vi "Expressions Example.vi"() -> ()   [LabVIEW 2022 SP3]
uses:
  Expressions/Expressions.lvlib
panel:
  out "error out":errorcluster
  in  "Expression":string(combo)="(a + b) * a - (c / b)"
  in  "f":bool=TRUE
  in  "e":bool
  in  "d":bool=TRUE
  in  "c":i32=-123
  in  "b":dbl=4.34
  in  "a":dbl=1.23
  out "Evaluated":dbl
  # "Instructions:\nEdit the Expression and run this VI to see the Evaluated result."
  # "The Expression statements are evaluated at run time.\nExpressions are first tokenized, parsed to postfix operations, then evaluated.\nAn expression can be nested in parentheses and consist of one or more operations,\nliterals, and/or variables. Supports either numerical expressions: (a + b * c) or \nboolean/conditional expressions: (a >= b or not c)."
  # "E.g. Numerical expression:    (a + b) * c"
  # "E.g. Boolean expression:    (d or e) and f"
  # "Variables"
  # "Supports:\nAND:          and | && | &\nOR:           or | '||' | '|'\nNOT:          not | !\nEQUAL:        ==\nNOT EQUAL:    !=\nLESS THAN:    <\nGREATER THAN: >\nLTE:          <=\nGTE:          >=\nPLUS:         +\nMINUS:        -\nMULTIPLY:     *\nDIVIDE:       /\nMODULUS:      %\nPARENTHESES:  (..)\nLITERAL:      Boolean | DBL | I32 | U32\nVARIABLE:    [A-Za-z_][A-Za-z0-9_]*\n  Note: Variables are referenced by name index."
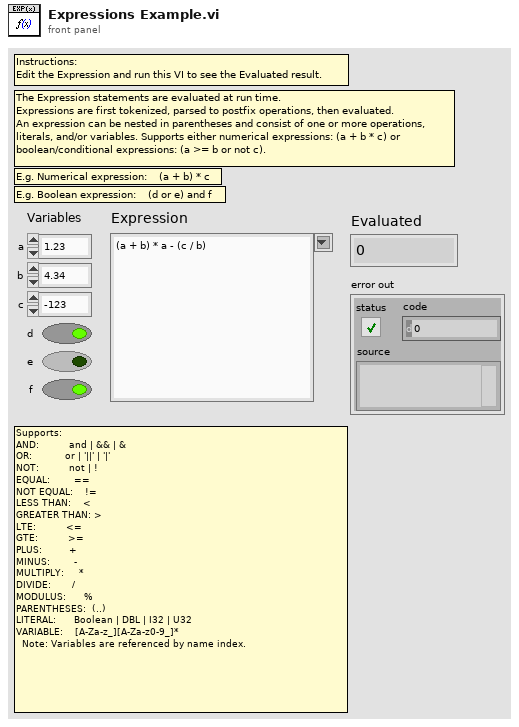
[diagram p1: front panel]
types:
  T1 = typedef "Expressions.lvlib/Expression.ctl" = cluster{"Types":T2[], "Values":dbl[]}
  T2 = typedef "Expressions.lvlib/Token Type.ctl" = enum8{"INVALID", "NOT", "AND", "OR", "EE", "NE", "LT", "GT", "LTE", "GTE", "PLUS", "MINUS", "MULTIPLY", "DIVIDE", "MODULUS", "LPAREN", "RPAREN", "LITERAL", "IDENTIFIER", "DEFINITION"}
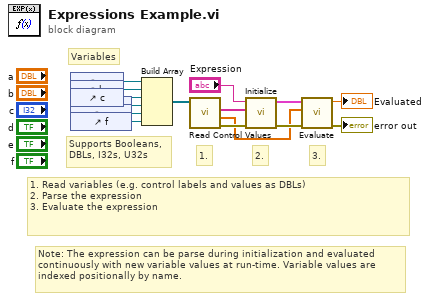
[diagram p0: block diagram]
diagram:
  # "Supports Booleans,\nDBLs, I32s, U32s"
  # "Note: The expression can be parse during initialization and evaluated\ncontinuously with new variable values at run-time. Variable values are\nindexed positionally by name."
  # "1. Read variables (e.g. control labels and values as DBLs)\n2. Parse the expression\n3. Evaluate the expression"
  # "3."
  # "2."
  # "1."
  # "Variables"
  n1 = control-ref of="a"() -> (w12:refnum<vi>)
  n2 = control-ref of="b"() -> (w11:refnum<vi>)
  n3 = control-ref of="c"() -> (w10:refnum<vi>)
  n4 = control-ref of="d"() -> (w9:refnum<vi>)
  n5 = control-ref of="e"() -> (w8:refnum<vi>)
  n6 = control-ref of="f"() -> (w7:refnum<vi>)
  n7 = Build Array(w12, w11, w10, w9, w8, w7) -> (w6:refnum<vi>[])
  n8 = call "Read Control Values.vi"("Control Refnums in"=w6) -> ("error out"=w14:errorcluster, "Variable Values"=w2:dbl[], "Variable Names"=w13:string[])  [unwired: 7 in, 1 out]
  n9 = call "Initialize.vi"("error in (no error)"=w14, "Variable Names"=w13, "Expression"="Expression") -> ("error out"=w3:errorcluster, "Expression"=w15:T1)  [unwired: 7 in]
  n10 = call "Evaluate.vi"("error in (no error)"=w3, "Variable Values"=w2, "Expression"=w15) -> ("error out"=→"error out":errorcluster, "Evaluated"=→"Evaluated":dbl)  [unwired: 7 in]
